vi "TdmsIcons_CloseFile.vi"(8 "error in (no error)":errorcluster, 11 "TdmsIn":refnum<k34>) -> (0 "error out":errorcluster, 3 "Path":path)   [LabVIEW 2014]
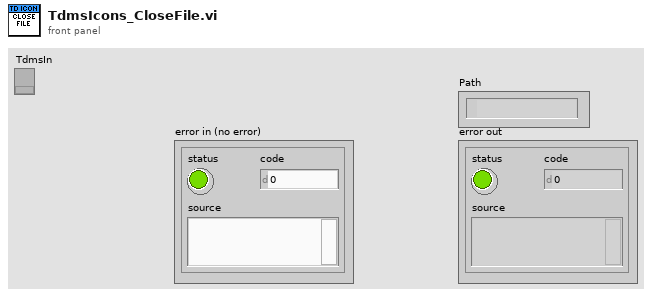
[diagram p1: front panel]
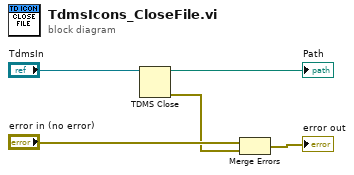
[diagram p0: block diagram]
diagram:
  n1 = TDMS Close(11:"TdmsIn") -> (0:w2:errorcluster, 3:→"Path":path)  [unwired: 1 in]
  n2 = Merge Errors("error in (no error)", w2) -> (→"error out":errorcluster)
